vi "InvokeMatlabMethod.vi"(8 "error in (no error)":errorcluster, 9 "ExpID":string, 10 "Method Name":string, 11 "Arguments":variant) -> (0 "error out":errorcluster)   [LabVIEW 2017]
uses:
  Types/MethodInvokeInfo.ctl
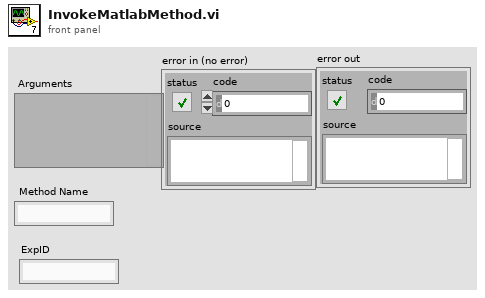
[diagram p1: front panel]
types:
  T1 = typedef "MethodInvokeInfo.ctl" = cluster{"Method Name":string, "Arguments":variant}
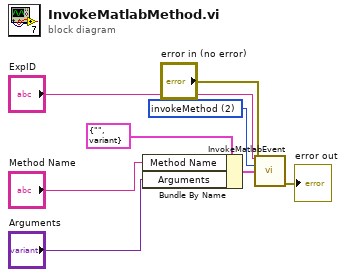
[diagram p0: block diagram]
diagram:
  w4 = u16 2 items=["[FromStringName]", "updateExpParameter", "invokeMethod"] ("Event")
  n1 = Bundle By Name(cluster=T1 {"Method Name"="", "Arguments"=variant}, "Method Name"="Method Name", "Arguments"="Arguments") -> (w6:T1)
  n2 = call "InvokeMatlabEvent.vi"("ExpID"="ExpID", "Event"=w4, "Data"=w6, "error in (no error)"="error in (no error)") -> ("error out"=→"error out":errorcluster)  [unwired: 11 in]
